vi "MainOCT TEst.vi"() -> ()   [LabVIEW 2017]
panel:
  out "finish time":timestamp
  out "start time":timestamp
  in  "Data Range":T1={"Z start (pxl)"=1, "Z length (pxl)"=400}
  in  "# Cscan":i32
  in  "Save Path":path=path "E:/Jiarui/1217test"
  out "error out":errorcluster
  in  "Objective":u16(ring)=1 items=["5X LKM05", "10X LKM10", "20X LKM20", "10X LSM02"]
  in  "ROI Parameters":T2={"ROI (mm)"={"X (mm)"=1.2, "Y (mm)"=1.2}, "Shift (mm)"={"Xshift (mm)"=0.0, "Yshift (mm)"=0.0}}
  in  "Scan Parameters":T3={"# Scan"={"#Ascan"=480, "#Bscan"=480}, "# Rpt"={"#ARpt"=1, "#BRpt"=1}, "Aline Rate"=2, "# Extra"={"# ARpt_extra"=5, "#Brtn_extra"=80}} {"Aline Rate" items=["76 KHz", "146 KHz", "76 KHz", "28 KHz", "10 KHz"]}
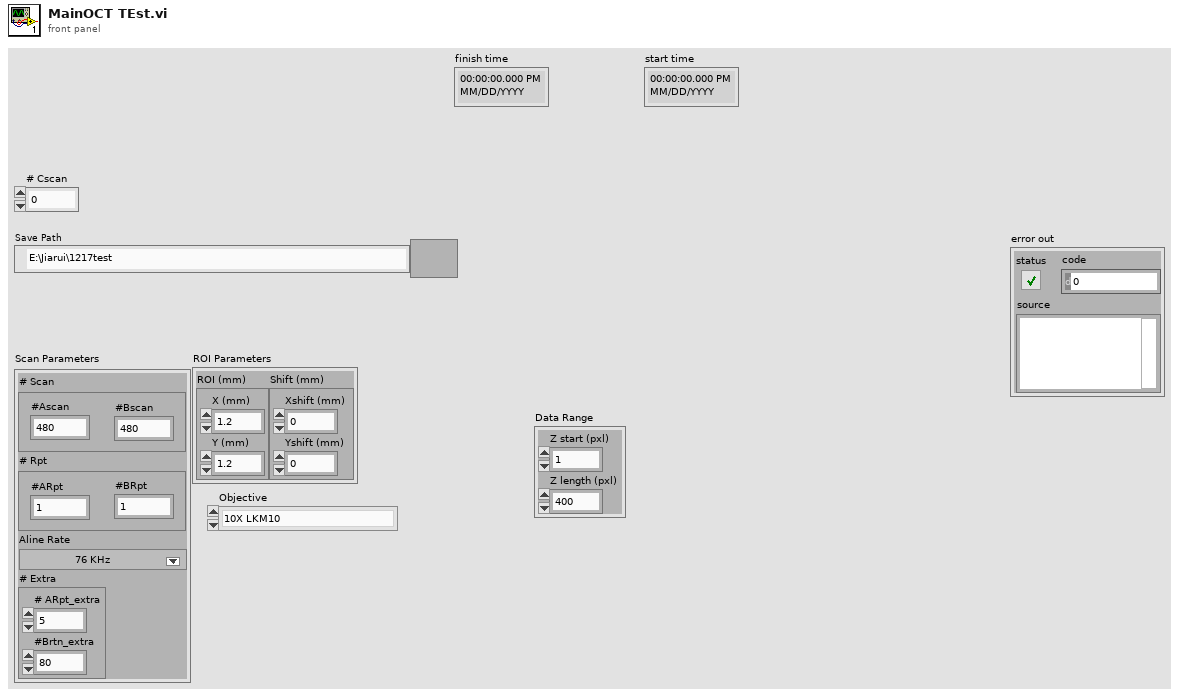
[diagram p1: front panel]
types:
  T1 = cluster{"Z start (pxl)":i32, "Z length (pxl)":i32}
  T2 = cluster{"ROI (mm)":cluster{"X (mm)":dbl, "Y (mm)":dbl}, "Shift (mm)":cluster{"Xshift (mm)":sgl, "Yshift (mm)":sgl}}
  T3 = cluster{"# Scan":cluster{"#Ascan":i32, "#Bscan":i32}, "# Rpt":cluster{"#ARpt":i32, "#BRpt":i32}, "Aline Rate":u16, "# Extra":cluster{"# ARpt_extra":i32, "#Brtn_extra":i32}}
  T4 = enum16{"Init", "Configure", "Configure Data", "Generate Scan Pattern", "Start Acquire Raw", "Start Acquire Data", "Acquire RAW", "Acquire Data", "Stop Acquire", "Uninit"}
  T5 = enum16{"Create", "Enqueue", "Dequeue", "Release"}
  T6 = cluster{"Image Index":i16, "Slice Index":i16, "#Cscan":i32, "nAT per B":i32, "nA per B":i32, "Brtn_extra/2":i32}
  T7 = cluster{"ROI (mm)":cluster{"X (mm)":sgl, "Y (mm)":sgl}, "Shift (mm)":cluster{"Xshift (mm)":sgl, "Yshift (mm)":sgl}}
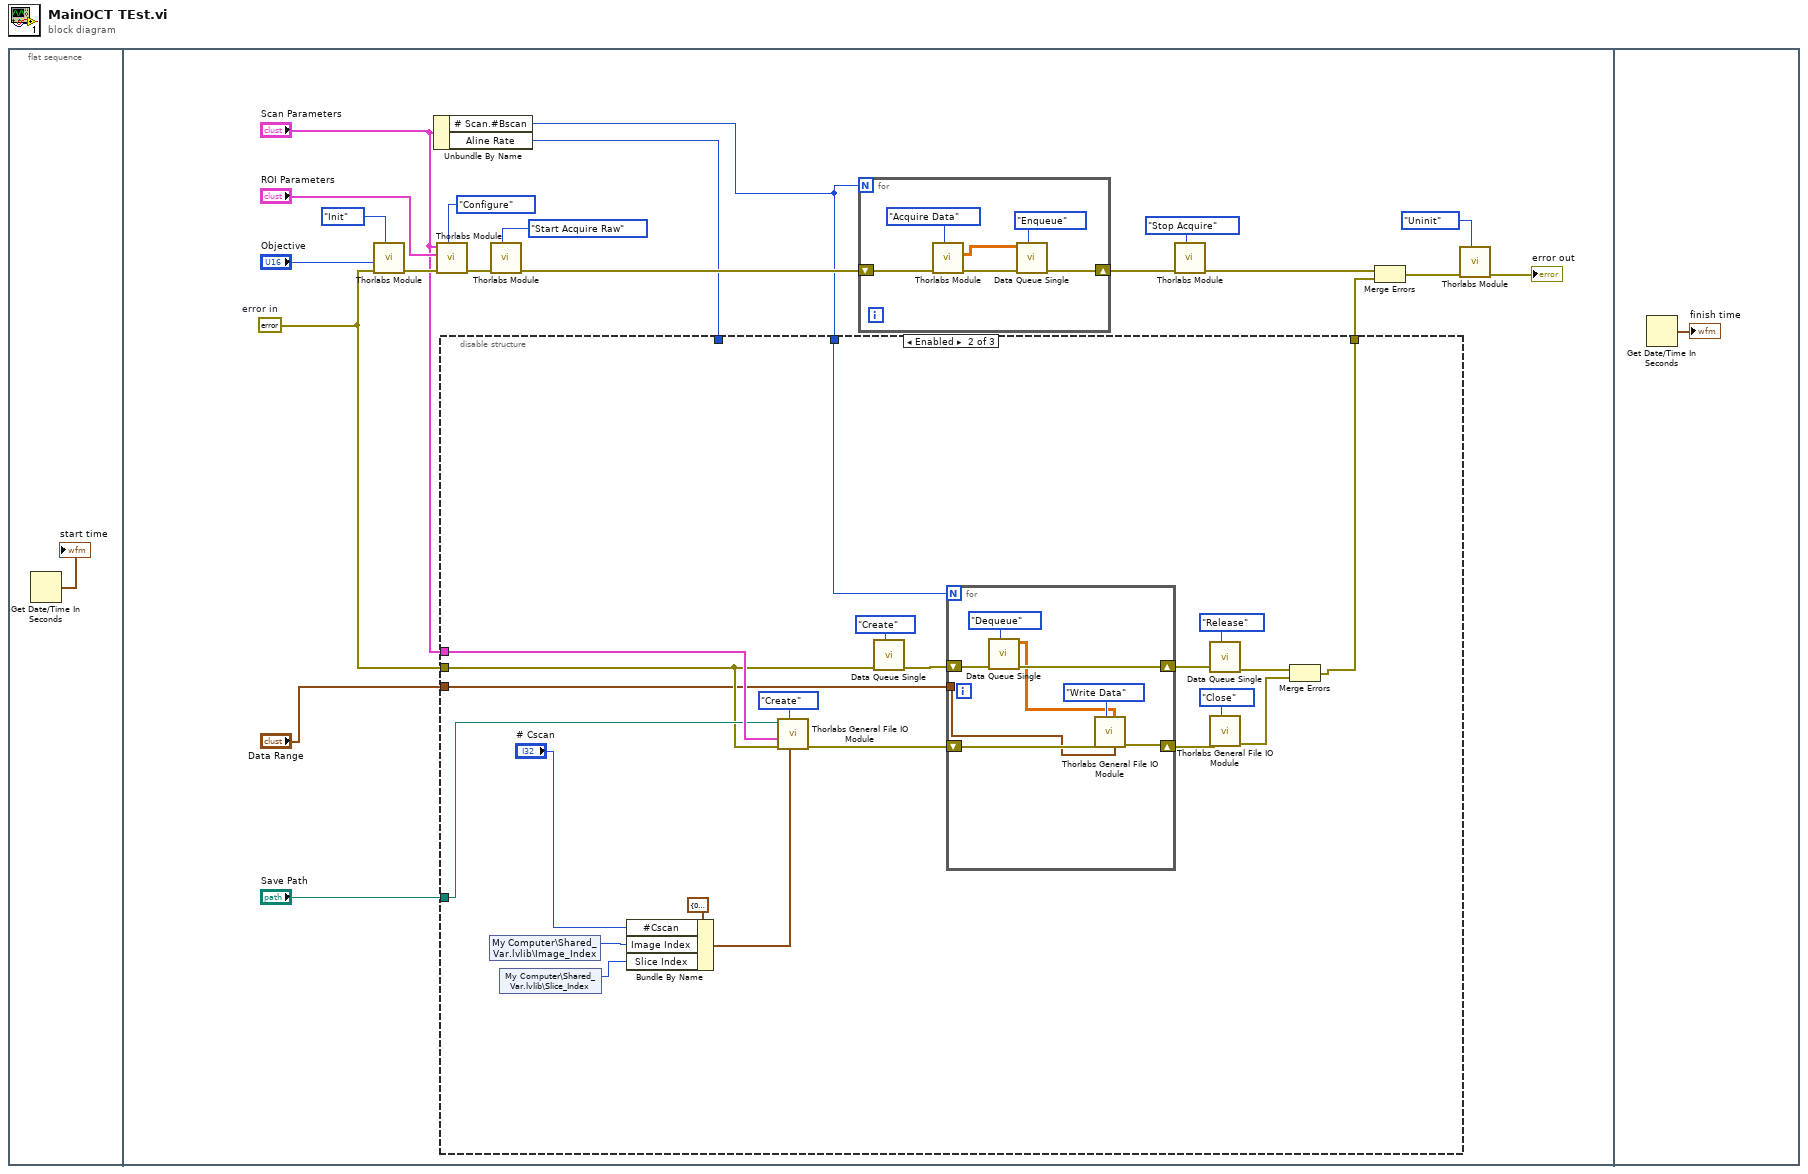
[diagram p0: block diagram]
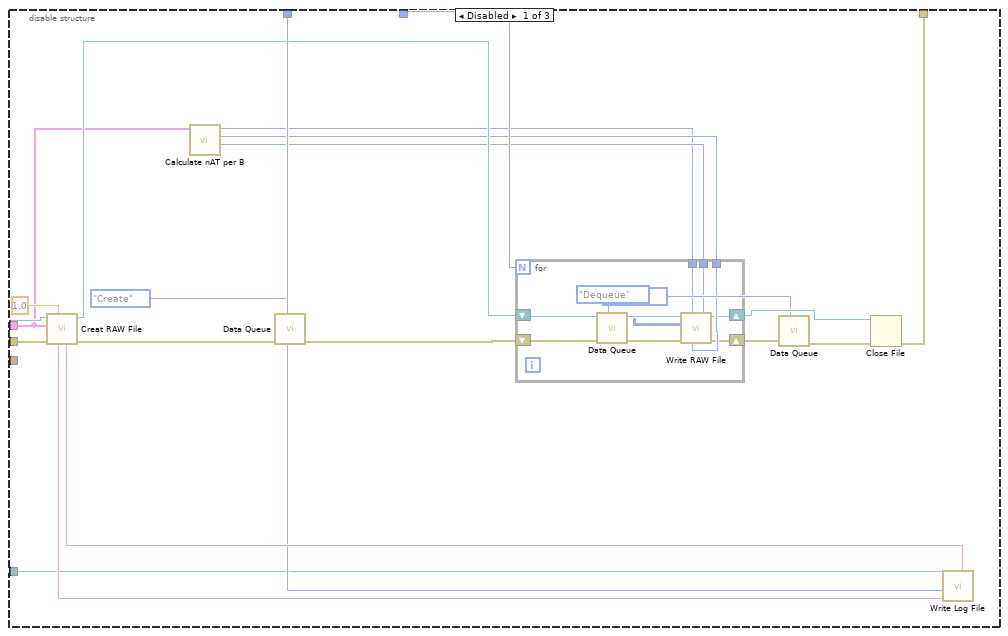
[diagram p2: hidden frame]
diagram:
  n1 = flat-sequence {
    frame #0 {
      n2 = Get Date/Time In Seconds() -> (seconds since 1Jan1904=→"start time":timestamp)
    }
    frame #1 {
      w14 = errorcluster {"status"=FALSE, "code"=0, "source"=""}  # error in
      n3 = call "Thorlabs Module.vi"("Actions"=T4."Init", "error in"=w14, "Objective"="Objective") -> ("error out"=w22:errorcluster)  [unwired: 6 in, 2 out]
      n4 = Unbundle By Name("Scan Parameters") -> ("# Scan.#Bscan"=w9:i32, "Aline Rate"=w12:u16)
      n5 = call "Thorlabs Module.vi"("Actions"=T4."Configure", "error in"=w22, "ROI Parameters"="ROI Parameters", "Scan Parameters"="Scan Parameters") -> ("error out"=w21:errorcluster)  [unwired: 5 in, 2 out]
      n6 = disable-structure shown="Enabled" {
        disable-tunnel: w14 -> [w46 w69 _]
        disable-tunnel: [w42 w71 _] -> w13
        disable-tunnel: w12 -> [w40 _ _]
        disable-tunnel: "Scan Parameters" -> [w29 w75 _]
        disable-tunnel: "Save Path" -> [w35 w70 _]
        disable-tunnel: w9 -> [w33 w76 _]
        disable-tunnel: "Data Range" -> [_ w61 _]
        frame Disabled {
          n7 = call "Creat RAW File.vi"("#Cscan"=1.0, "error in"=w46, "Scan Parameters"=w29, "Save Path"=w35) -> ("error out"=w47:errorcluster, "refnum out"=w34:refnum<file>, "Save Name"=w45:string, "Scan Parameter"=w44:string)  [unwired: 4 in]
          n8 = call "Calculate nAT per B.vi"("Scan Parameters"=w29) -> ("nA per B"=w32:i32, "Brtn_extra/2"=w31:i32, "nAT per B"=w30:i32)  [unwired: 8 in]
          n9 = call "Data Queue.vi"("Action"=T5."Create", "error in (no error)"=w47) -> ("error out"=w36:errorcluster)  [unwired: 8 in, 1 out]
          n10 = for {
            N: w33 -> [_]
            tunnel: w32 -> [w60]
            tunnel: w31 -> [w59]
            tunnel: w30 -> [w58]
            shift-right: [w56] -> w38
            shift-left: w36 -> [w54]
            shift-right: [w57] -> w41
            shift-left: w34 -> [w52]
            n11 = call "Data Queue.vi"("Action"=T5."Dequeue", "error in (no error)"=w54) -> ("error out"=w53:errorcluster, "Data Out"=w51:u16[][])  [unwired: 8 in]
            n12 = call "Write RAW File.vi"("nA per B"=w60, "Brtn_extra/2"=w59, "nAT per B"=w58, "error constant"=w53, "Data In"=w51, "refnum in"=w52) -> ("error out"=w56:errorcluster, "refnum out"=w57:refnum<file>)  [unwired: 4 in]
          }
          n13 = call "Data Queue.vi"("Action"=T5."Release", "error in (no error)"=w38) -> ("error out"=w43:errorcluster)  [unwired: 8 in, 1 out]
          n14 = Close File(refnum=w41, error in=w43) -> (error out=w42:errorcluster)  [unwired: 1 out]
          n15 = call "Write Log File.vi"("Save Name"=w45, "Scan Parameter"=w44, "Aline Rate"=w40, "Save Path"=w35) -> ("ROI Parameters"=w49:T7, "Objective"=w50:u16)  [unwired: 6 in]
        }
        frame Enabled {
          n16 = shared-variable "My Computer\\Shared_Var.lvlib\\Image_Index"() -> (w67:i16)  [unwired: 1 in, 1 out]
          n17 = shared-variable "My Computer\\Shared_Var.lvlib\\Slice_Index"() -> (w66:i16)  [unwired: 1 in, 1 out]
          n18 = Bundle By Name(cluster=T6 {"Image Index"=0, "Slice Index"=0, "#Cscan"=0, "nAT per B"=0, "nA per B"=0, "Brtn_extra/2"=0} ("Imaging Parameters"), "#Cscan"="# Cscan", "Image Index"=w67, "Slice Index"=w66) -> (w65:T6)
          n19 = call "Thorlabs General File IO Module.vi"("Imaging Parameters"=w65, "Actions"=enum16{"Create", "Write", "Write Data", "Close"}."Create", "error in"=w69, "Scan Parameters"=w75, "Save Path"=w70) -> ("error out"=w74:errorcluster)  [unwired: 4 in, 2 out]
          n20 = call "Data Queue Single.vi"("Action"=T5."Create", "error in (no error)"=w69) -> ("error out"=w77:errorcluster)  [unwired: 8 in, 1 out]
          n21 = for {
            N: w76 -> [_]
            shift-right: [w85] -> w79
            shift-left: w77 -> [w88]
            shift-right: [w86] -> w73
            shift-left: w74 -> [w87]
            tunnel: w61 -> [w82]
            n22 = call "Data Queue Single.vi"("Action"=T5."Dequeue", "error in (no error)"=w88) -> ("error out"=w85:errorcluster, "Data Out"=w83:sgl[][])  [unwired: 8 in]
            n23 = call "Thorlabs General File IO Module.vi"("Data Range"=w82, "Data In"=w83, "Actions"=enum16{"Create", "Write", "Write Data", "Close"}."Write Data", "error in"=w87) -> ("error out"=w86:errorcluster)  [unwired: 5 in, 2 out]
          }
          n24 = call "Data Queue Single.vi"("Action"=T5."Release", "error in (no error)"=w79) -> ("error out"=w81:errorcluster)  [unwired: 8 in, 1 out]
          n25 = call "Thorlabs General File IO Module.vi"("Actions"=enum16{"Create", "Write", "Write Data", "Close"}."Close", "error in"=w73) -> ("error out"=w72:errorcluster)  [unwired: 7 in, 2 out]
          n26 = Merge Errors(w81, w72) -> (w71:errorcluster)
        }
        frame Disabled {
        }
      }
      n27 = call "Thorlabs Module.vi"("Actions"=T4."Start Acquire Raw", "error in"=w21) -> ("error out"=w20:errorcluster)  [unwired: 7 in, 2 out]
      n28 = for {
        N: w9 -> [_]
        shift-right: [w26] -> w11
        shift-left: w20 -> [w28]
        n29 = call "Thorlabs Module.vi"("Actions"=T4."Acquire Data", "error in"=w28) -> ("error out"=w27:errorcluster, "Data Out"=w23:sgl[][])  [unwired: 7 in, 1 out]
        n30 = call "Data Queue Single.vi"("Action"=T5."Enqueue", "error in (no error)"=w27, "Data In"=w23) -> ("error out"=w26:errorcluster)  [unwired: 7 in, 1 out]
      }
      n31 = call "Thorlabs Module.vi"("Actions"=T4."Stop Acquire", "error in"=w11) -> ("error out"=w19:errorcluster)  [unwired: 7 in, 2 out]
      n32 = Merge Errors(w19, w13) -> (w18:errorcluster)
      n33 = call "Thorlabs Module.vi"("Actions"=T4."Uninit", "error in"=w18) -> ("error out"=→"error out":errorcluster)  [unwired: 7 in, 2 out]
    }
    frame #2 {
      n34 = Get Date/Time In Seconds() -> (seconds since 1Jan1904=→"finish time":timestamp)
    }
  }
